vi "SEK2020v1VI6TamanhodoEspaçoVazio.vi"(8 "Parâmetros":T1={"Azul Max EV3 Cor"=17, "Azul Min EV3 Cor"=0, "Verde Max EV3 Cor"=6.0, "Verde Min EV3 Cor"=0.0, "Vermelho Max Ev3 Cor"=0, "Vermelho Min EV3 Cor"=0, "Chão EV3 Cor"=0.0, "Branco Max EV3 Cor"=0.0, "Branco Min EV3 Cor"=0.0, "Preto Max EV3 Cor"=0.0, "Preto Min EV3 Cor"=0.0, "Distância Tubulação"=0.0, "Distância Frontal"=0.0, "Amarelo Max EV3 Cor"=0.0, "Amarelo Min EV3 Cor"=0.0, "Distância Lateral"=0.0, "90°"=0.0, "180°"=0.0, "Seguidor de Linha"=0.0}, 9 "d-e":i32, 10 "NXT/EV3":T2) -> (1 "Tamanho do tubo":dbl, 2 "NXT/EV3 2":T2)   [LabVIEW 2016]
uses:
  <vilib>/NXT/Block Support/NXT_OutputPort.ctl
  <vilib>/NXT/NXTIO Xnodes/AddressXNode/NXTIOAddress.xnode
  <vilib>/NXT/Dual Mode Library/Motors/ResetMotor.vi
  <vilib>/NXT/Block Support/NXT_InputPort.ctl
  <vilib>/NXT/Dual Mode Library/Sensors/EV3_Gyro_Angle.vi
  <vilib>/NXT/Dual Mode Library/Sensors/EV3_Ultrasonic_CM.vi
  <vilib>/NXT/Dual Mode Library/Motors/Rotation.vi
  <vilib>/NXT/NXTIO Xnodes/NXTIOXNode/NXTIO.xnode
  <vilib>/NXT/Subs/LVHSConnector.ctl
  <vilib>/NXT/LegoClasses/BrickReference/BrickReference.lvclass
  <vilib>/NXT/NXTIO Xnodes/NXTIONodeSubVIs/NXTStopMotors.vi
  <vilib>/NXT/Hardware/Plugins/Open Port/OpenPortAddress.ctl
  <vilib>/NXT/Dual Mode Library/Sensors/Touch_Pressed.vi
  <vilib>/NXT/Dual Mode Library/Sensors/EV3_Color_Reflect.vi
  <vilib>/NXT/Dual Mode Library/Sensors/EV3_Gyro_Reset.vi
panel:
  # "Sensor EV3 Cor"
  # "Sensor Ultrassônico"
  # "Sensor Giroscópio"
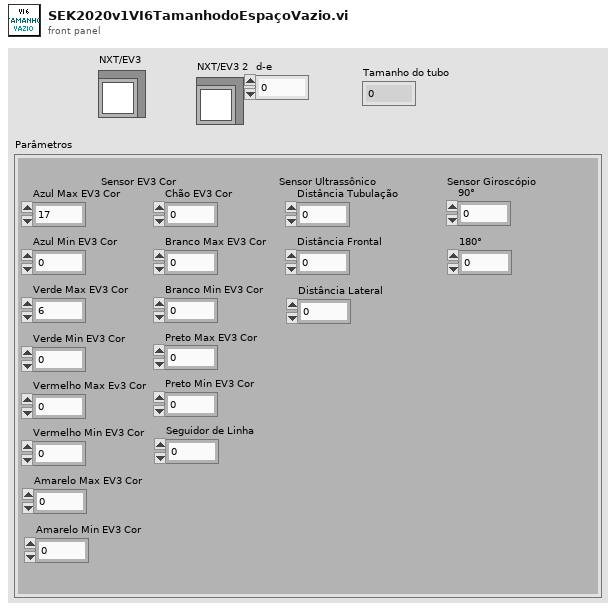
[diagram p1: front panel]
types:
  T1 = cluster{"Azul Max EV3 Cor":i32, "Azul Min EV3 Cor":i32, "Verde Max EV3 Cor":dbl, "Verde Min EV3 Cor":dbl, "Vermelho Max Ev3 Cor":i32, "Vermelho Min EV3 Cor":i32, "Chão EV3 Cor":sgl, "Branco Max EV3 Cor":sgl, "Branco Min EV3 Cor":sgl, "Preto Max EV3 Cor":sgl, "Preto Min EV3 Cor":sgl, "Distância Tubulação":sgl, "Distância Frontal":sgl, "Amarelo Max EV3 Cor":dbl, "Amarelo Min EV3 Cor":dbl, "Distância Lateral":sgl, "90°":sgl, "180°":sgl, "Seguidor de Linha":dbl}
  T2 = typedef "LVHSConnector.ctl" = refnum<class "BrickReference.lvclass">
  T3 = typedef "NXT_InputPort.ctl" = u32
  T4 = typedef "NXT_OutputPort.ctl" = u8
  T5 = typedef "OpenPortAddress.ctl" = i32
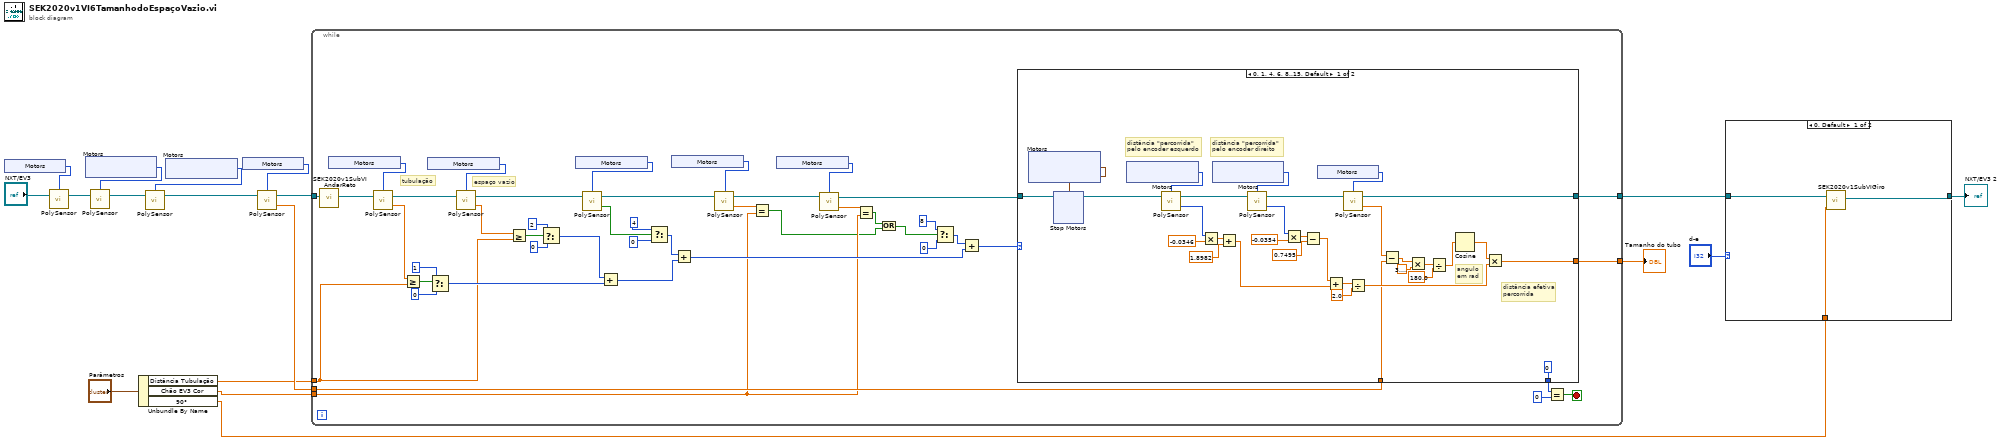
[diagram p0: block diagram]
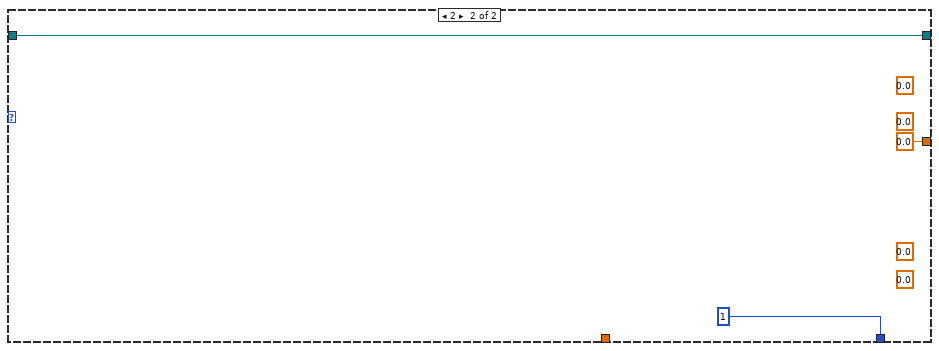
[diagram p3: hidden frame]
diagram:
  n1 = xnode "Motors"() -> ("Sensor"=w15:T3)
  n2 = call-poly <vilib>:"PolySensor.vi"("NXT/EV3"="NXT/EV3", "Port (Port 1)"=w15) -> ("NXT/EV3"=w16:T2)  [unwired: 2 in]
  n3 = xnode "Motors"() -> ("Motor"=w18:T4)
  n4 = call-poly <vilib>:"PolySensor.vi"("NXT/EV3"=w16, "Port (All Ports)"=w18) -> ("NXT/EV3"=w17:T2)  [unwired: 2 in]
  n5 = Unbundle By Name("Parâmetros") -> ("Distância Tubulação"=w4:sgl, "Chão EV3 Cor"=w3:sgl, "90°"=w1:sgl)
  n6 = xnode "Motors"() -> ("Motor"=w14:T4)
  n7 = call-poly <vilib>:"PolySensor.vi"("NXT/EV3"=w17, "Port (All Ports)"=w14) -> ("NXT/EV3"=w11:T2)  [unwired: 2 in]
  n8 = xnode "Motors"() -> ("Sensor"=w10:T3)
  n9 = call-poly <vilib>:"PolySensor.vi"("NXT/EV3"=w11, "Port (Port 1)"=w10) -> ("Degrees"=w9:sgl, "NXT/EV3"=w12:T2)  [unwired: 1 in]
  n10 = while {
    tunnel: w12 -> [w42]
    tunnel: w9 -> [w41]
    tunnel: [w40] -> w2
    tunnel: [w39] -> w7
    tunnel: w4 -> [w34]
    tunnel: w3 -> [w22]
    stop <- w46 stop-if-true
    # "espaço vazio"
    # "tubulação"
    n11 = call "SEK2020v1SubVIAndarReto.vi"("NXT/EV3"=w42) -> ("NXT/EV3 2"=w43:T2)  [unwired: 9 in]
    n12 = xnode "Motors"() -> ("Sensor"=w37:T5)
    n13 = call-poly <vilib>:"PolySensor.vi"("NXT/EV3"=w43, "Port (Port 1)"=w37) -> ("Centimeters"=w61:sgl, "NXT/EV3"=w63:T2)  [unwired: 1 in]
    n14 = Greater Or Equal?(x=w61, y=w34) -> (x >= y?=w59:bool)
    n15 = xnode "Motors"() -> ("Sensor"=w36:T5)
    n16 = Select(t=1, s=w59, f=0) -> (s? t:f=w50:i32)
    n17 = call-poly <vilib>:"PolySensor.vi"("NXT/EV3"=w63, "Port (Port 1)"=w36) -> ("Centimeters"=w60:sgl, "NXT/EV3"=w62:T2)  [unwired: 1 in]
    n18 = Greater Or Equal?(x=w60, y=w34) -> (x >= y?=w56:bool)
    n19 = Select(t=2, s=w56, f=0) -> (s? t:f=w49:i32)
    n20 = xnode "Motors"() -> ("Sensor"=w35:T5)
    n21 = call-poly <vilib>:"PolySensor.vi"("NXT/EV3"=w62, "Port (Port 1)"=w35) -> ("Yes / No"=w53:bool, "NXT/EV3"=w38:T2)  [unwired: 1 in]
    n22 = Add(x=w49, y=w50) -> (x+y=w47:i32)
    n23 = Select(t=4, s=w53, f=0) -> (s? t:f=w48:i32)
    n24 = xnode "Motors"() -> ("Sensor"=w33:T5)
    n25 = Add(x=w48, y=w47) -> (x+y=w28:i32)
    n26 = call-poly <vilib>:"PolySensor.vi"("NXT/EV3"=w38, "Port (Port 1)"=w33) -> ("Scaled Value"=w32:sgl, "NXT/EV3"=w24:T2)  [unwired: 1 in]
    n27 = Equal?(x=w32, y=w22) -> (x = y?=w20:bool)
    n28 = xnode "Motors"() -> ("Sensor"=w25:T5)
    n29 = call-poly <vilib>:"PolySensor.vi"("NXT/EV3"=w24, "Port (Port 1)"=w25) -> ("Scaled Value"=w26:sgl, "NXT/EV3"=w23:T2)  [unwired: 1 in]
    n30 = Equal?(x=w26, y=w22) -> (x = y?=w21:bool)
    n31 = Or(x=w21, y=w20) -> (x .or. y?=w19:bool)
    n32 = Select(t=8, s=w19, f=0) -> (s? t:f=w29:i32)
    n33 = Add(x=w29, y=w28) -> (x+y=w27:i32)
    n34 = case shown="0, 1, 4, 6, 8..15, Default" w27 {
      tunnel: w23 -> [w77 w112]
      tunnel: [0 1] -> w44
      tunnel: w41 -> [w78 _]
      tunnel: [w82 w112] -> w39
      tunnel: [w81 0.0] -> w40
      frame 0, 1, 4, 6, 8..15, Default {
        # "angulo \nem rad"
        # "distância efetiva\npercorrida"
        # "distância \"percorrida\" \npelo encoder direito"
        # "distância \"percorrida\" \npelo encoder esquerdo"
        n35 = xnode "Motors"() -> ("Motor"=w75:cluster{"Port":T4, "Port":T4})
        n36 = xnode "Stop Motors"("Motors"=w75, "NXT/EV3"=w77) -> ("NXT/EV3"=w76:T2)
        n37 = xnode "Motors"() -> ("Motor"=w97:T4)
        n38 = call-poly <vilib>:"PolySensor.vi"("NXT/EV3"=w76, "Port (Port A)"=w97) -> ("Angle of Rotation"=w94:i32, "NXT/EV3"=w95:T2)  [unwired: 1 in]
        n39 = Multiply(x=w94, y=-0.0346) -> (x*y=w92:dbl)
        n40 = xnode "Motors"() -> ("Motor"=w96:T4)
        n41 = Add(x=w92, y=1.8982) -> (x+y=w80:dbl)
        n42 = call-poly <vilib>:"PolySensor.vi"("NXT/EV3"=w95, "Port (Port A)"=w96) -> ("Angle of Rotation"=w90:i32, "NXT/EV3"=w83:T2)  [unwired: 1 in]
        n43 = Multiply(x=w90, y=-0.0354) -> (x*y=w88:dbl)
        n44 = Subtract(x=w88, y=0.7495) -> (x-y=w79:dbl)
        n45 = xnode "Motors"() -> ("Sensor"=w99:T3)
        n46 = Add(x=w79, y=w80) -> (x+y=w86:dbl)
        n47 = call-poly <vilib>:"PolySensor.vi"("NXT/EV3"=w83, "Port (Port 1)"=w99) -> ("Degrees"=w98:sgl, "NXT/EV3"=w82:T2)  [unwired: 1 in]
        n48 = Divide(x=w86, y=2.0) -> (x/y=w84:dbl)
        n49 = Subtract(x=w98, y=w78) -> (x-y=w73:sgl)
        n50 = Multiply(x=w73, y=3.141592653589793) -> (x*y=w71:dbl)
        n51 = Divide(x=w71, y=180.0) -> (x/y=w69:dbl)
        n52 = Cosine(x=w69) -> (cos(x)=w74:dbl)
        n53 = Multiply(x=w74, y=w84) -> (x*y=w81:dbl)
      }
      frame 2 {
        (unwired) sgl 0.0
        (unwired) sgl 0.0
        (unwired) 0.0
        (unwired) 0.0
      }
    }
    n54 = Equal?(x=w44, y=0) -> (x = y?=w46:bool)
  }
  "Tamanho do tubo" <- w2
  n55 = case shown="0, Default" "d-e" {
    tunnel: w7 -> [w115 w116]
    tunnel: [w114 w116] -> w6
    tunnel: w1 -> [w113 _]
    frame 0, Default {
      n56 = call "SEK2020v1SubVIGiro.vi"("ANGULO"=w113, "NXT/EV3"=w115) -> ("NXT/EV3 2"=w114:T2)  [unwired: 7 in]
    }
    frame 1 {
    }
  }
  "NXT/EV3 2" <- w6
